vi "offset.vi"(1 "offset":dbl, 2 "x":dbl) -> (0 "y":dbl)   [LabVIEW 2019]
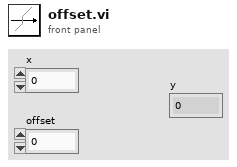
[diagram p1: front panel]
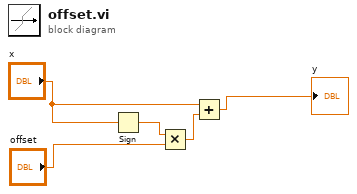
[diagram p0: block diagram]
diagram:
  n1 = Sign(1:"x") -> (0:w5:dbl)
  n2 = Multiply(x=w5, y="offset") -> (x*y=w2:dbl)
  n3 = Add(x="x", y=w2) -> (x+y=→"y":dbl)
